vi "ReadTiffPage_I16_text.vi"(0 "TIFF file":T2 {"BigTiff,Endian" items=["Big-Endian"=0, "Native"=1, "Little-Endian"=2, "BigTiff-Big-Endian"=256, "Bigtiff,Native"=257, "Biftiff,Littleendian"=258]}, 2 "IFDoffset":i64, 3 "error in":errorcluster) -> (6 "TIFF file out":T2 {"BigTiff,Endian" items=["Big-Endian"=0, "Native"=1, "Little-Endian"=2, "BigTiff-Big-Endian"=256, "Bigtiff,Native"=257, "Biftiff,Littleendian"=258]}, 7 "16-bit pixmap":i16[][](array[numeric]), 8 "string":string, 9 "Next offset":i64, 10 "error out":errorcluster)   [LabVIEW 2011]
uses:
  IFD.ctl
  GetTagValue_U64.vi
  GetTagValues_U8s.vi
panel:
  out "Byte-Reihenfolge (0:Big-Endian, Netzwerkreihenfolge)":T1(ring)=enum."native, host order"
  out "Bytes":u64
  out "Bits":u32
  out "BildOffset":u64
  out "Width":u64
  out "Length":u64
  out "Directory Entries":T3[](array[typedef])
  out "IFDs":u16
  # "seems to work!"
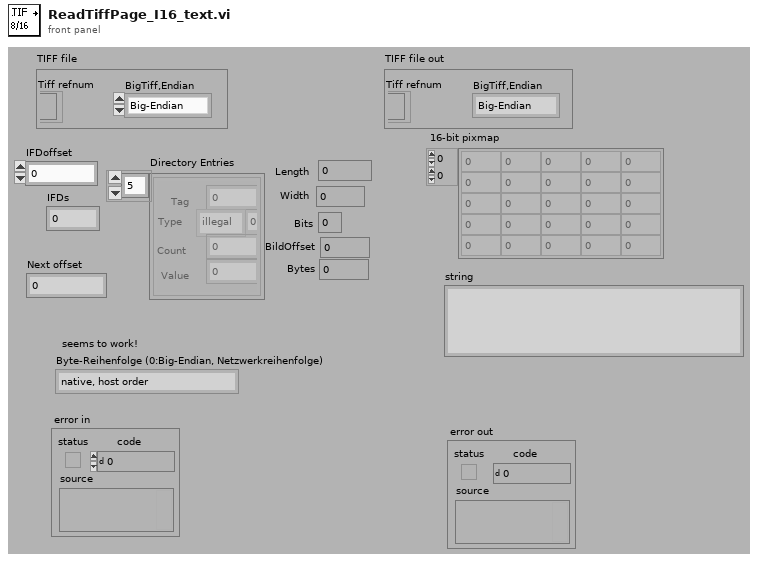
[diagram p1: front panel]
types:
  T1 = enum16{"big-endian, network order", "native, host order", "little-endian"}
  T2 = cluster{"Tiff refnum":refnum<file>, "BigTiff,Endian":u16}
  T3 = typedef "IFD.ctl" = cluster{"Tag":u16, "Type":enum16{"illegal", "Byte", "Ascii", "Short", "Long", "Rational", "SByte", "Undefined", "SShort", "SLong", "SRational 2xSLong", "Float 4byte", "Double 8Byte", "No13", "No14", "No15", "U64", "I64", "U64-IFD8"}, "Count":u64, "Value":u64}
  T4 = cluster{"Tag":u16, "Type":enum16{"illegal", "Byte", "Ascii", "Short", "Long", "Rational", "SByte", "Undefined", "SShort", "SLong", "SRational 2xSLong", "Float 4byte", "Double 8Byte"}, "Count":u32, "Value":u32}
  T5 = cluster{"Tag":u16, "Type":enum16{"illegal", "Byte", "Ascii", "Short", "Long", "Rational", "SByte", "Undefined", "SShort", "SLong", "SRational 2xSLong", "Float 4byte", "Double 8Byte"}, "Count":u32, "Value":u32}[]
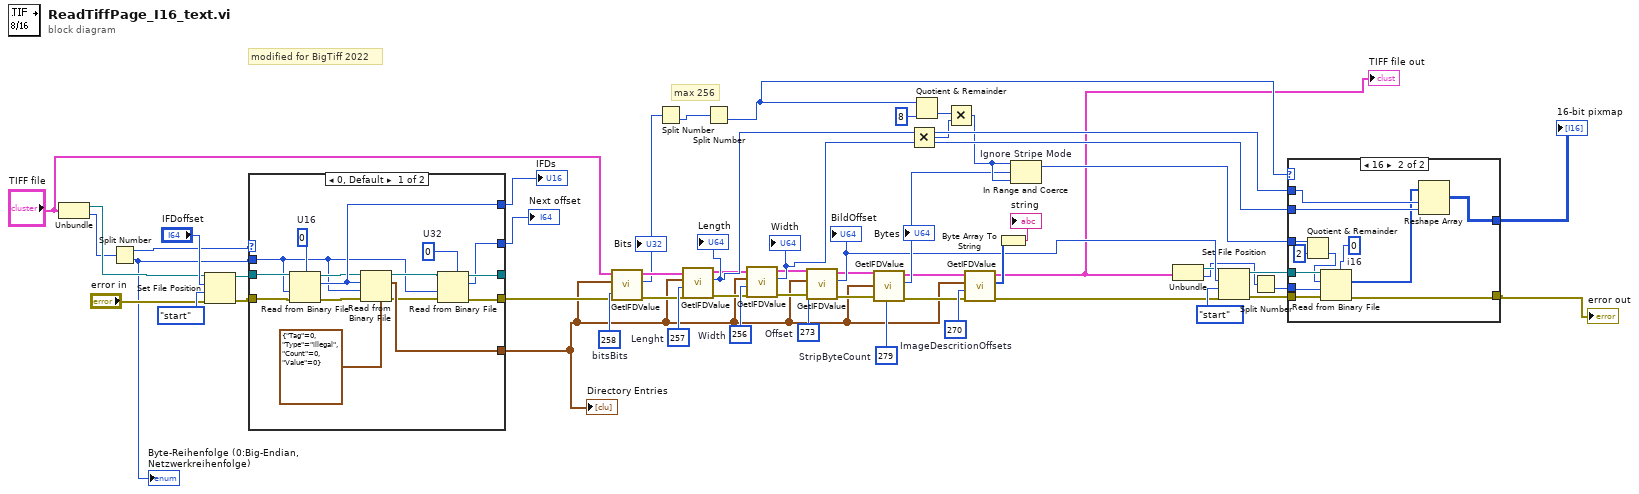
[diagram p0: block diagram]
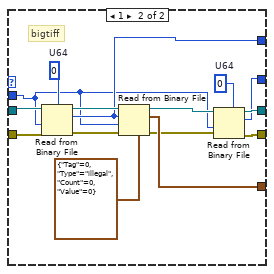
[diagram p2: hidden frame]
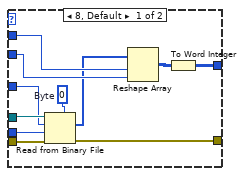
[diagram p3: hidden frame]
diagram:
  w35 = u16 270  # ImageDescritionOffsets
  w45 = u16 256  # Width
  w51 = u16 258  # bitsBits
  w44 = u16 279  # StripByteCount
  w47 = u16 257  # Lenght
  w46 = u16 273  # Offset
  # "modified for BigTiff 2022"
  # "max 256"
  n1 = Unbundle("TIFF file") -> ("Tiff refnum"=w48:refnum<file>, "BigTiff,Endian"=w15:u16)
  n2 = Split Number(x=w15) -> (hi(x)=w5:u8, lo(x)=w6:u8)
  "Byte-Reihenfolge (0:Big-Endian, Netzwerkreihenfolge)" <- w6
  n3 = Set File Position(offset (in bytes) (0)="IFDoffset", refnum=w48, from (0:start)=enum16{"start", "end", "current"}."start" ("pos mode (0:2)"), error in="error in") -> (refnum out=w7:refnum<file>, error out=w8:errorcluster)
  n4 = case shown="0, Default" w5 {
    tunnel: [w68 w78] -> w2
    tunnel: w8 -> [w67 w80]
    tunnel: w7 -> [w66 w79]
    tunnel: [w59 w73] -> _
    tunnel: [w58 w75] -> w4
    tunnel: [w63 w77] -> w1
    tunnel: w6 -> [w55 w72]
    tunnel: [w57 w70] -> w3
    frame 0, Default {
      w56 = u32 0  # U32
      w69 = u16 0  # U16
      n5 = Read from Binary File(5:w69, 8:w67, 9:w55, 11:w66) -> (0:w64:errorcluster, 2:w68:u16, 3:w65:refnum<file>)  [unwired: 3 out]
      n6 = Read from Binary File(5:T4 {"Tag"=0, "Type"=enum."illegal", "Count"=0, "Value"=0} ("Cluster"), 8:w64, 9:w55, 10:w68, 11:w65) -> (0:w61:errorcluster, 2:w63:T5, 3:w60:refnum<file>)  [unwired: 2 out]
      n7 = Read from Binary File(5:w56, 8:w61, 9:w55, 11:w60) -> (0:w58:errorcluster, 2:w57:u32, 3:w59:refnum<file>)  [unwired: 3 out]
    }
    frame 1 {
      w71 = u64 0  # U64
      w84 = u64 0  # U64
      # "bigtiff"
      n8 = Read from Binary File(5:w84, 8:w80, 9:w72, 11:w79) -> (0:w82:errorcluster, 2:w78:u64, 3:w83:refnum<file>)  [unwired: 3 out]
      n9 = Read from Binary File(5:T3 {"Tag"=0, "Type"=enum."illegal", "Count"=0, "Value"=0} ("Cluster"), 8:w82, 9:w72, 10:w78, 11:w83) -> (0:w76:errorcluster, 2:w77:T3[], 3:w74:refnum<file>)  [unwired: 2 out]
      n10 = Read from Binary File(5:w71, 8:w76, 9:w72, 11:w74) -> (0:w75:errorcluster, 2:w70:u64, 3:w73:refnum<file>)  [unwired: 3 out]
    }
  }
  "IFDs" <- w2
  "Directory Entries" <- w1
  "Next offset" <- w3
  n11 = call-poly "GetIFDValue.vi"("error in (no error)"=w4, "Tag Code"=w51, "Directory Entries"=w1, "TIFF file"="TIFF file") -> ("error out"=w31:errorcluster, "Single Value"=w13:u64, "TIFF file out"=w33:T2)  [unwired: 3 out]
  "Bits" <- w13
  n12 = Split Number(x=w13) -> (lo(x)=w14:u32)  [unwired: 1 out]
  n13 = call-poly "GetIFDValue.vi"("error in (no error)"=w31, "Tag Code"=w47, "Directory Entries"=w1, "TIFF file"=w33) -> ("error out"=w30:errorcluster, "Single Value"=w43:u64, "TIFF file out"=w32:T2)  [unwired: 3 out]
  "Length" <- w43
  n14 = Split Number(x=w14) -> (lo(x)=w12:u16)  [unwired: 1 out]
  n15 = call-poly "GetIFDValue.vi"("error in (no error)"=w30, "Tag Code"=w45, "Directory Entries"=w1, "TIFF file"=w32) -> ("error out"=w26:errorcluster, "Single Value"=w42:u64, "TIFF file out"=w28:T2)  [unwired: 3 out]
  "Width" <- w42
  n16 = call-poly "GetIFDValue.vi"("error in (no error)"=w26, "Tag Code"=w46, "Directory Entries"=w1, "TIFF file"=w28) -> ("error out"=w25:errorcluster, "Single Value"=w29:u64, "TIFF file out"=w27:T2)  [unwired: 3 out]
  "BildOffset" <- w29
  n17 = call-poly "GetIFDValue.vi"("error in (no error)"=w25, "Tag Code"=w44, "Directory Entries"=w1, "TIFF file"=w27) -> ("error out"=w24:errorcluster, "Single Value"=w37:u64, "TIFF file out"=w23:T2)  [unwired: 3 out]
  "Bytes" <- w37
  n18 = Multiply(x=w43, y=w42) -> (x*y=w40:u64)
  n19 = Quotient & Remainder(x=w12, y=u32 8) -> (floor(x/y)=w39:u32)  [unwired: 1 out]
  n20 = Multiply(x=w39, y=w40) -> (x*y=w38:u64)
  n21 = call-poly "GetIFDValue.vi"("error in (no error)"=w24, "Tag Code"=w35, "Directory Entries"=w1, "TIFF file"=w23) -> ("error out"=w9:errorcluster, "Byte array"=w34:u8[], "TIFF file out"=w10:T2)  [unwired: 3 out]
  "TIFF file out" <- w10
  n22 = Byte Array To String(unsigned byte array=w34) -> (string=→"string":string)
  n23 = In Range and Coerce "Ignore Stripe Mode"(upper limit=w38, x=w37, lower limit=w38) -> (coerced(x)=w17:u64)  [unwired: 1 out]
  n24 = Unbundle(w10) -> ("Tiff refnum"=w21:refnum<file>, "BigTiff,Endian"=w16:u16)
  n25 = Set File Position(offset (in bytes) (0)=w29, refnum=w21, from (0:start)=enum16{"start", "end", "current"}."start" ("pos mode (0:2)"), error in=w9) -> (refnum out=w20:refnum<file>, error out=w19:errorcluster)
  n26 = Split Number(x=w16) -> (lo(x)=w11:u8)  [unwired: 1 out]
  n27 = case shown="16" w12 {
    tunnel: w43 -> [w95 w107]
    tunnel: w42 -> [w94 w106]
    tunnel: [w85 w105] -> w50
    tunnel: w20 -> [w92 w104]
    tunnel: w19 -> [w91 w103]
    tunnel: [w90 w97] -> w18
    tunnel: w17 -> [w87 w101]
    tunnel: w11 -> [w86 w102]
    frame 8, Default {
      w88 = u8 0  # Byte
      n28 = Read from Binary File(5:w88, 8:w91, 9:w86, 10:w87, 11:w92) -> (0:w90:errorcluster, 2:w89:u8[])  [unwired: 3 out]
      n29 = Reshape Array(w89, w95, w94) -> (w93:u8[][])
      n30 = To Word Integer(number=w93) -> (16bit integer=w85:i16[][])
    }
    frame 16 {
      w98 = i16 0  # i16
      n31 = Quotient & Remainder(x=w101, y=u32 2) -> (floor(x/y)=w99:u64)  [unwired: 1 out]
      n32 = Read from Binary File(5:w98, 8:w103, 9:w102, 10:w99, 11:w104) -> (0:w97:errorcluster, 2:w96:i16[])  [unwired: 3 out]
      n33 = Reshape Array(w96, w107, w106) -> (w105:i16[][])
    }
  }
  "error out" <- w18
  "16-bit pixmap" <- w50
